vi "Commit HSDIO.vi"(11 "Semiconductor Module Context":T1) -> (0 "error out":errorcluster)   [LabVIEW 2013]
uses:
  <vilib>/NI_TestStand_SemiconductorModule/NI_TestStand_Semiconductor_Module.lvlibp/PinMap/General/SemiconductorModuleContext.ctl
  <instrlib>/niHSDIO/niHSDIO.llb/niHSDIO Commit Dynamic.vi
  <instrlib>/niHSDIO/niHSDIO.llb/niHSDIO Commit Static.vi
  <vilib>/NI_TestStand_SemiconductorModule/NI_TestStand_Semiconductor_Module.lvlibp
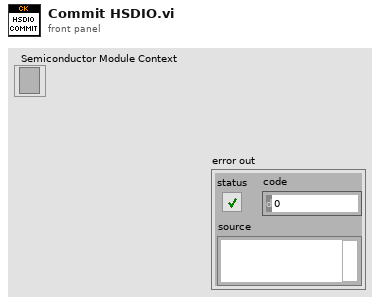
[diagram p1: front panel]
types:
  T1 = typedef "NI_TestStand_Semiconductor_Module.lvlibp/SemiconductorModuleContext.ctl" = refnum<k7>
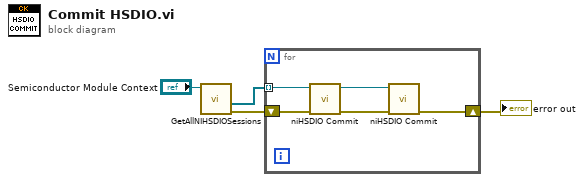
[diagram p0: block diagram]
diagram:
  n1 = call <vilib>:"GetAllNIHSDIOSessions.vi"("Semiconductor Module Context"="Semiconductor Module Context") -> ("error out"=w3:errorcluster, "Generation Sessions"=w2:refnum<k15>[])  [unwired: 7 in, 2 out]
  n2 = for {
    tunnel: w2 -> [w8] mode=indexing
    shift-right: [w5] -> w1
    shift-left: w3 -> [w9]
    n3 = call-poly <instrlib>:"niHSDIO Commit.vi"("error in (no error)"=w9, "instrument handle"=w8) -> ("error out"=w7:errorcluster, "instrument handle out"=w6:refnum<k15>)  [unwired: 8 in]
    n4 = call-poly <instrlib>:"niHSDIO Commit.vi"("error in (no error)"=w7, "instrument handle"=w6) -> ("error out"=w5:errorcluster)  [unwired: 8 in, 1 out]
  }
  "error out" <- w1
